vi "US distance.vi"() -> ()   [LabVIEW 2020]
panel:
  out "Waveform Chart 2":dynamicdata(graph)
  out "Numeric":dbl
  in  "stop":bool
  out "Waveform Chart":dbl(graph)
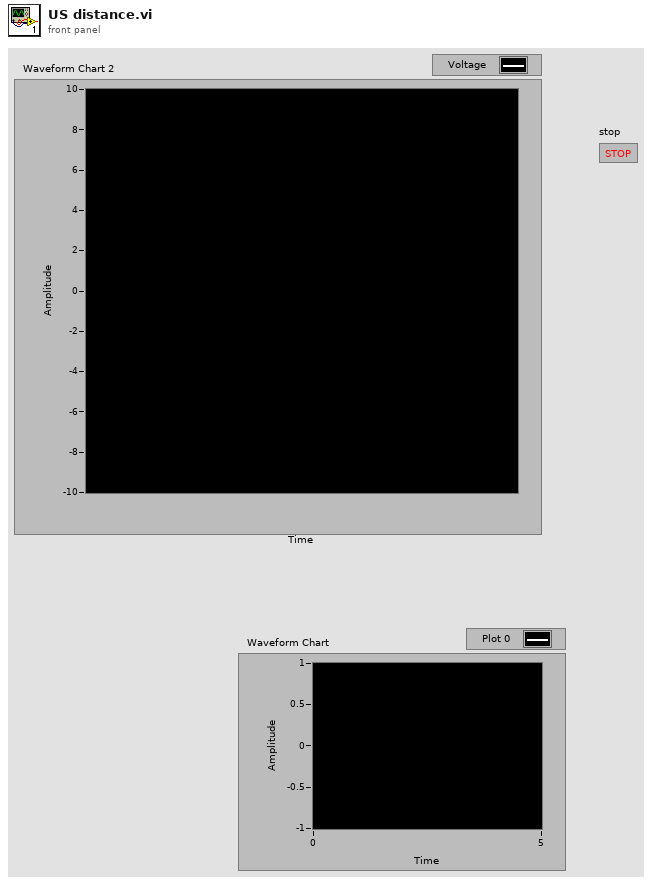
[diagram p1: front panel]
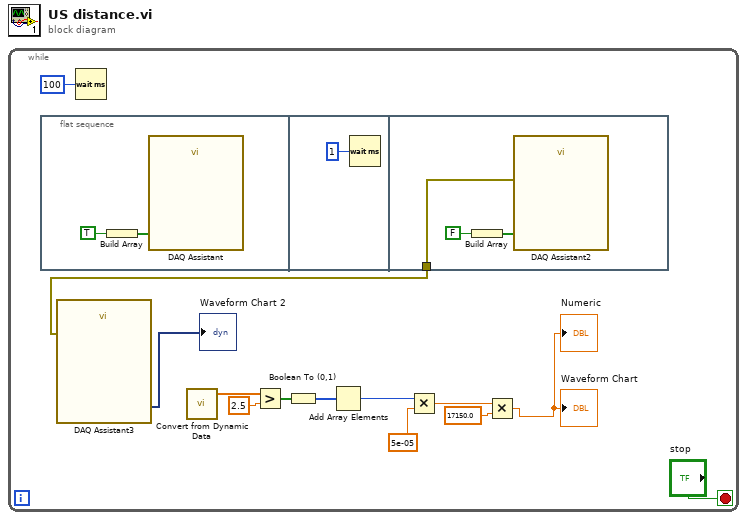
[diagram p0: block diagram]
diagram:
  n1 = while {
    stop <- "stop" stop-if-true
    n2 = flat-sequence {
      tunnel: [w17] -> w1
      frame #0 {
        n3 = Build Array(TRUE) -> (w14:bool[])
        n4 = call "DAQ Assistant"("data"=w14) -> ()  [unwired: 17 in, 2 out]
      }
      frame #1 {
        n5 = Wait (ms)(milliseconds to wait=u32 1) -> ()  [unwired: 1 out]
      }
      frame #2 {
        n6 = Build Array(FALSE) -> (w18:bool[])
        n7 = call "DAQ Assistant2"("data"=w18) -> ("error out"=w17:errorcluster)  [unwired: 17 in, 1 out]
      }
    }
    n8 = call "DAQ Assistant3"("error in"=w1) -> ("data"=→"Waveform Chart 2":dynamicdata)  [unwired: 16 in, 2 out]
    n9 = Wait (ms)(milliseconds to wait=u32 100) -> ()  [unwired: 1 out]
    n10 = call "Convert from Dynamic Data"() -> ("Array"=w9:dbl[])  [unwired: 4 in]
    n11 = Greater?(x=w9, y=2.5) -> (0:w8:bool[])
    n12 = Boolean To (0,1)(Boolean=w8) -> (0, 1=w7:i16[])
    n13 = Add Array Elements(numeric array=w7) -> (sum=w6:i16)
    n14 = Multiply(x=w6, y=5e-05) -> (x*y=w5:dbl)
    n15 = Multiply(x=w5, y=17150.0) -> (x*y=→"Numeric" →"Waveform Chart":dbl)
  }
